vi "I64 to String.vi"(8 "Error In":errorcluster, 10 "I64":i64, 11 "String in":string) -> (0 "Error Out":errorcluster, 3 "String out":string)   [LabVIEW 2011, in "Tinkerforge.lvlib" / "Device.lvclass"]
doc: "This VI converts a numeric I64 string into a binary little-endian I64."
uses:
  Device.lvclass
  IP Connection/IP Connection.lvclass
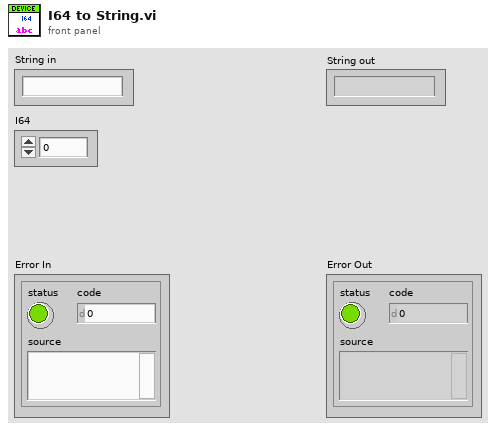
[diagram p1: front panel]
types:
  T1 = enum16{"big-endian, network order", "native, host order", "little-endian"}
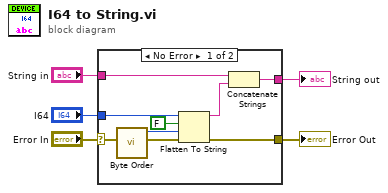
[diagram p0: block diagram]
diagram:
  n1 = case shown="No Error" "Error In" {
    selector: "Error In" -> [w13 w15]
    tunnel: "String in" -> [w8 w14]
    tunnel: [w11 w15] -> w3
    tunnel: [w6 w14] -> w2
    tunnel: "I64" -> [w9 _]
    frame No Error {
      n2 = call "Byte Order.vi"() -> ("byte order (2:little-endian)"=w12:T1)  [unwired: 11 in]
      n3 = Flatten To String(anything=w9, prepend array or string size? (T)=FALSE, byte order (0:big-endian, network order)=w12, error in (no error)=w13) -> (data string=w7:string, error out=w11:errorcluster)  [unwired: 1 out]
      n4 = Concatenate Strings(w8, w7) -> (w6:string)
    }
    frame Error {
    }
  }
  "Error Out" <- w3
  "String out" <- w2
